vi "Next Max Velocity.vi"(1 "Forward":bool, 2 "dt":dbl, 3 "Constrains":T1, 4 "Velocity":dbl) -> (0 "Next Max Velocity":dbl)   [LabVIEW 2015]
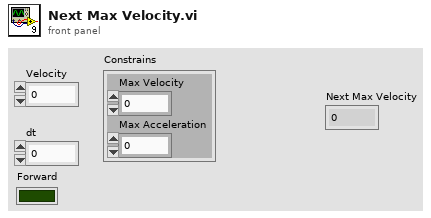
[diagram p1: front panel]
types:
  T1 = cluster{"Max Velocity":dbl, "Max Acceleration":dbl}
  T2 = typedef "Control 1.ctl" = dbl
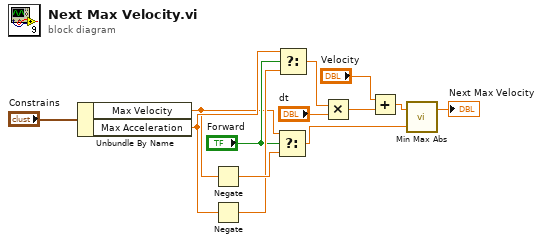
[diagram p0: block diagram]
diagram:
  n1 = Unbundle By Name("Constrains") -> ("Max Velocity"=w3:dbl, "Max Acceleration"=w10:dbl)
  n2 = Negate(x=w3) -> (-x=w12:dbl)
  n3 = Negate(x=w10) -> (-x=w11:dbl)
  n4 = Select(t=w3, s="Forward", f=w12) -> (s? t:f=w1:dbl)
  n5 = Select(t=w10, s="Forward", f=w11) -> (s? t:f=w7:dbl)
  n6 = Multiply(x=w7, y="dt") -> (x*y=w5:dbl)
  n7 = Add(x="Velocity", y=w5) -> (x+y=w4:dbl)
  n8 = call "Min Max Abs.vi"("b"=w1, "a"=w4) -> ("MinAbs(a,b)"=→"Next Max Velocity":T2)  [unwired: 1 out]
